vi "XLP80_Datalog_Globals.vi"() -> ()   [LabVIEW 2021]
panel:
  in  "Datalog":refnum<vi>
  out "Filename":path
  # "ms"
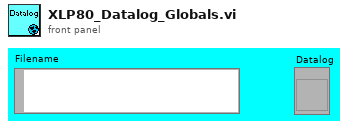
[diagram p1: front panel]
diagram:
